vi "Initialise All Modbus Devices.vi"(8 "error in (no error)":errorcluster, 11 "Data Cluster in":T1 {"Flexi-Flow Devices"."Control State"."Control Mode" items=["Bus/RS232"=0, "FLOW-BUS slave"=2, "Valve close"=3, "Controller idle"=4, "Setpoint 100%"=7, "Valve fully open"=8, "Calibration mode"=9, "Setpoint 0%"=12, "RS232"=18, "Valve steering"=20, "Valve safe state"=22]}) -> (0 "error out":errorcluster, 3 "Data Cluster out":T1 {"Flexi-Flow Devices"."Control State"."Control Mode" items=["Bus/RS232"=0, "FLOW-BUS slave"=2, "Valve close"=3, "Controller idle"=4, "Setpoint 100%"=7, "Valve fully open"=8, "Calibration mode"=9, "Setpoint 0%"=12, "RS232"=18, "Valve steering"=20, "Valve safe state"=22]})   [LabVIEW 2025]
uses:
  phlair-shared-libraries/Modbus Flexi-Flow API/Bronkhorst Flexi-Flow ModbusTCP API.lvlib
  phlair-shared-libraries/Modbus Flexi-Flow API/Control Function Values--enum.ctl
  Modbus Flexi-Flow Controls--cluster.ctl
  FlexiFlowInterface.lvlib
  <vilib>/Plasmionique/MB Master/MB_Master_TCP/MB_Master_TCP.lvclass
  Modbus Flexi-Flow Measure State--cluster.ctl
  Modbus Flexi-Flow State--cluster.ctl
  Module Data--cluster.ctl
  phlair-shared-libraries/Modbus Flexi-Flow API/Control Mode--enum.ctl
  Device Type--enum.ctl
  Modbus TCP Connection Settings--cluster.ctl
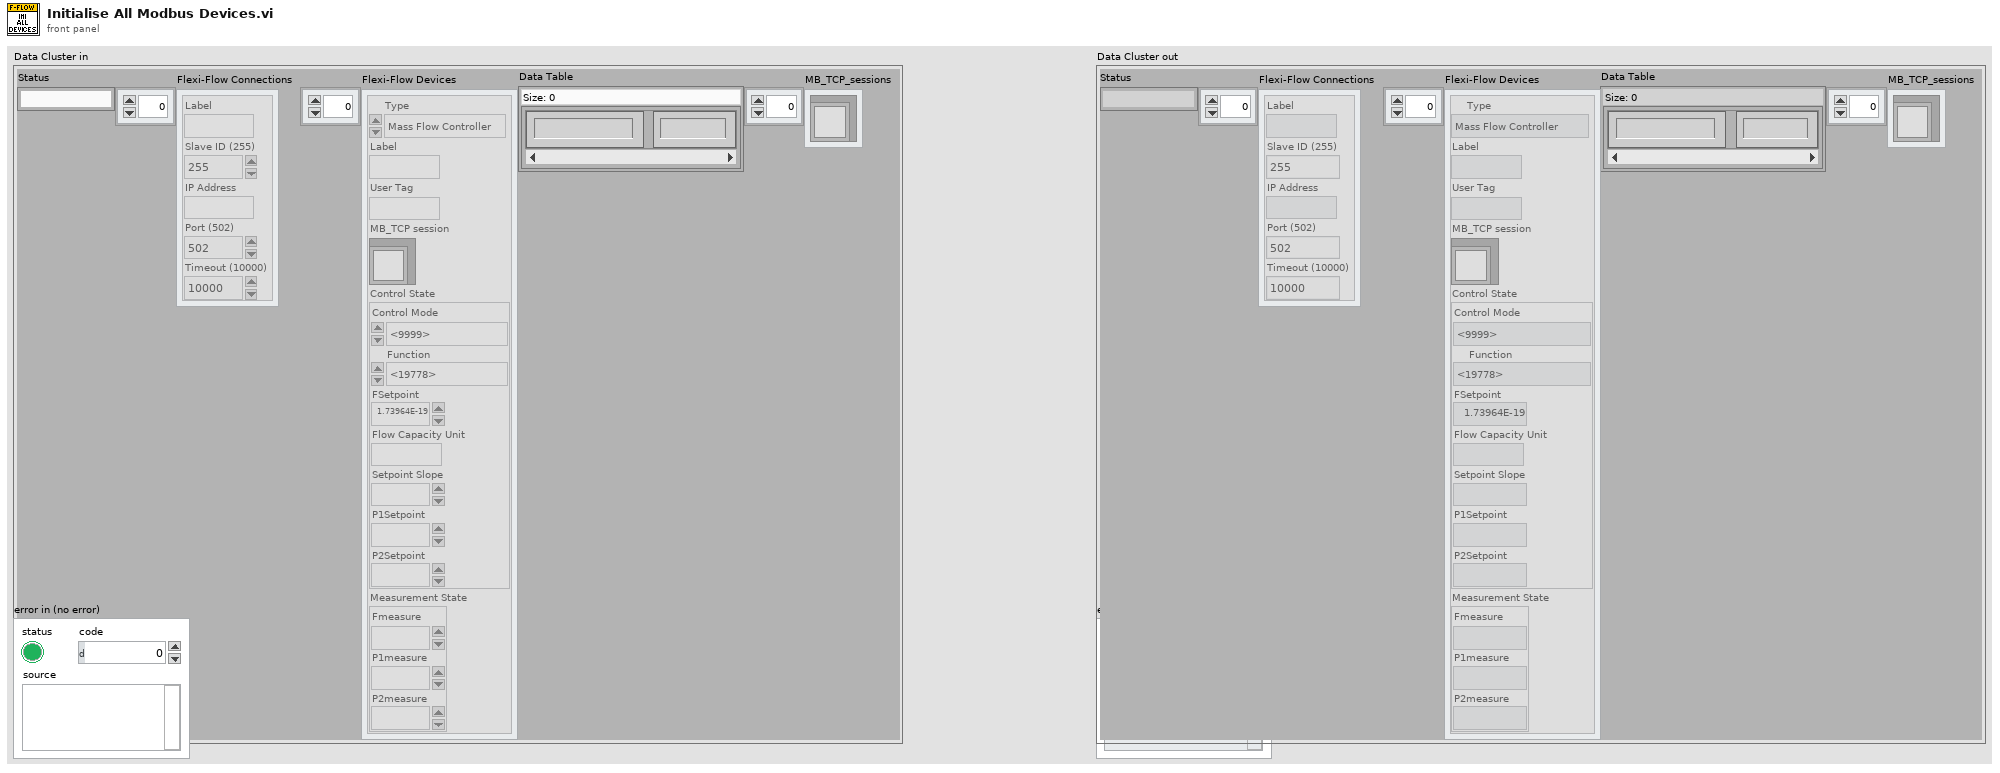
[diagram p1: front panel]
types:
  T1 = typedef "FlexiFlowInterface.lvlib/Module Data--cluster.ctl" = cluster{"Status":string, "Flexi-Flow Connections":T2[], "Flexi-Flow Devices":T3[], "Data Table":map{string, dbl}, "MB_TCP_sessions":refnum<class "MB_Master_TCP.lvclass">[]}
  T2 = typedef "FlexiFlowInterface.lvlib/Modbus TCP Connection Settings--cluster.ctl" = cluster{"Label":string, "Slave ID (255)":u8, "IP Address":string, "Port (502)":u16, "Timeout (10000)":i32}
  T3 = typedef "FlexiFlowInterface.lvlib/Modbus Flexi-Flow State--cluster.ctl" = cluster{"Type":T4, "Label":string, "User Tag":string, "MB_TCP session":refnum<class "MB_Master_TCP.lvclass">, "Control State":T5, "Measurement State":T8}
  T4 = typedef "FlexiFlowInterface.lvlib/Device Type--enum.ctl" = enum16{"Mass Flow Controller", "Mass Flow Meter"}
  T5 = typedef "FlexiFlowInterface.lvlib/Modbus Flexi-Flow Controls--cluster.ctl" = cluster{"Control Mode":T6, "Function":T7, "FSetpoint":sgl, "Flow Capacity Unit":string, "Setpoint Slope":u16, "P1Setpoint":sgl, "P2Setpoint":sgl}
  T6 = typedef "Bronkhorst Flexi-Flow ModbusTCP API.lvlib/Control Mode--enum.ctl" = u16
  T7 = typedef "Bronkhorst Flexi-Flow ModbusTCP API.lvlib/Control Function Values--enum.ctl" = enum16{"Flow", "Upstream pressure", "Downstream pressure", "Flow with upstream pressure limit", "Flow with downstream pressure limit", "Upstream pressure with flow limit", "Downstream pressure with flow limit"}
  T8 = typedef "FlexiFlowInterface.lvlib/Modbus Flexi-Flow Measure State--cluster.ctl" = cluster{"Fmeasure":dbl, "P1measure":sgl, "P2measure":sgl}
  T9 = typedef "FlexiFlowInterface.lvlib/Modbus Flexi-Flow State--cluster.ctl" = cluster{"MB_TCP session":refnum<class "MB_Master_TCP.lvclass">, "Control State":T10, "Measurement State":T8}
  T10 = typedef "FlexiFlowInterface.lvlib/Modbus Flexi-Flow Controls--cluster.ctl" = cluster{"Function":T7, "Control SP":sgl}
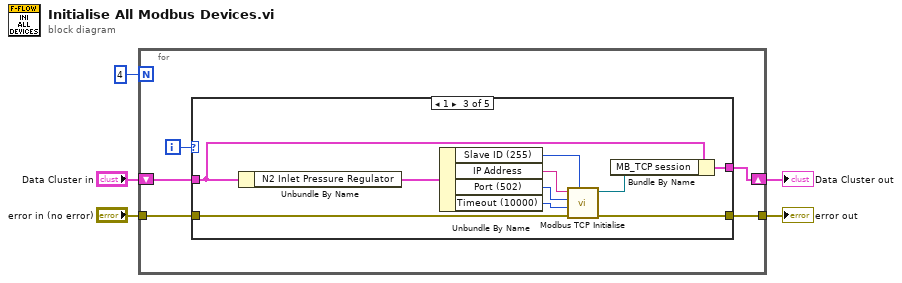
[diagram p0: block diagram]
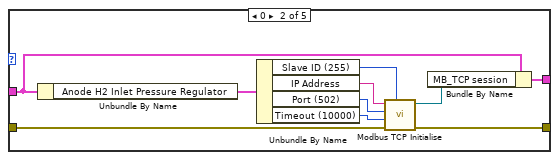
[diagram p3: hidden frame]
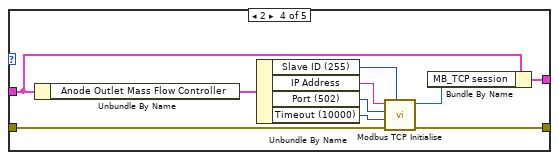
[diagram p4: hidden frame]
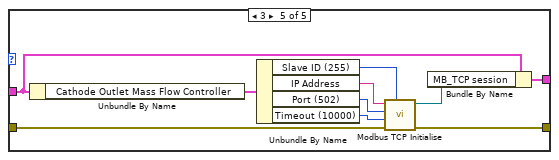
[diagram p5: hidden frame]
diagram:
  n1 = for {
    N: 4 -> [_]
    shift-right: [w9] -> w4
    shift-left: "Data Cluster in" -> [w8]
    tunnel: "error in (no error)" -> [w7]
    tunnel: [w10] -> w5
    i -> [w6]
    n2 = case shown="1" w6 {
      tunnel: [w12 w21 w31 w41 w51] -> w10
      tunnel: [w11 w20 w30 w40 w50] -> w9
      tunnel: w8 -> [w11 w17 w24 w34 w44]
      tunnel: w7 -> [w12 w19 w29 w39 w49]
      frame Default {
      }
      frame 0 {
        n3 = Unbundle By Name(w17) -> ("Anode H2 Inlet Pressure Regulator"=w18:T9)
        n4 = Unbundle By Name(w18) -> ("Slave ID (255)"=w13:u8, "IP Address"=w16:string, "Port (502)"=w15:u16, "Timeout (10000)"=w14:i32)
        n5 = call "Modbus TCP Initialise.vi"("Slave ID (255)"=w13, "error in (no error)"=w19, "Timeout (10000)"=w14, "Port (502)"=w15, "IP Address"=w16) -> ("error out"=w21:errorcluster, "MB_TCP session"=w22:refnum<class "MB_Master_TCP.lvclass">)  [unwired: 5 in]
        n6 = Bundle By Name(cluster=w17, "MB_TCP session"=w22) -> (w20:T1)
      }
      frame 1 {
        n7 = Unbundle By Name(w24) -> ("N2 Inlet Pressure Regulator"=w23:T9)
        n8 = Unbundle By Name(w23) -> ("Slave ID (255)"=w26:u8, "IP Address"=w25:string, "Port (502)"=w27:u16, "Timeout (10000)"=w28:i32)
        n9 = call "Modbus TCP Initialise.vi"("Slave ID (255)"=w26, "error in (no error)"=w29, "Timeout (10000)"=w28, "Port (502)"=w27, "IP Address"=w25) -> ("error out"=w31:errorcluster, "MB_TCP session"=w32:refnum<class "MB_Master_TCP.lvclass">)  [unwired: 5 in]
        n10 = Bundle By Name(cluster=w24, "MB_TCP session"=w32) -> (w30:T1)
      }
      frame 2 {
        n11 = Unbundle By Name(w34) -> ("Anode Outlet Mass Flow Controller"=w33:T9)
        n12 = Unbundle By Name(w33) -> ("Slave ID (255)"=w36:u8, "IP Address"=w35:string, "Port (502)"=w37:u16, "Timeout (10000)"=w38:i32)
        n13 = call "Modbus TCP Initialise.vi"("Slave ID (255)"=w36, "error in (no error)"=w39, "Timeout (10000)"=w38, "Port (502)"=w37, "IP Address"=w35) -> ("error out"=w41:errorcluster, "MB_TCP session"=w42:refnum<class "MB_Master_TCP.lvclass">)  [unwired: 5 in]
        n14 = Bundle By Name(cluster=w34, "MB_TCP session"=w42) -> (w40:T1)
      }
      frame 3 {
        n15 = Unbundle By Name(w44) -> ("Cathode Outlet Mass Flow Controller"=w43:T9)
        n16 = Unbundle By Name(w43) -> ("Slave ID (255)"=w46:u8, "IP Address"=w45:string, "Port (502)"=w47:u16, "Timeout (10000)"=w48:i32)
        n17 = call "Modbus TCP Initialise.vi"("Slave ID (255)"=w46, "error in (no error)"=w49, "Timeout (10000)"=w48, "Port (502)"=w47, "IP Address"=w45) -> ("error out"=w51:errorcluster, "MB_TCP session"=w52:refnum<class "MB_Master_TCP.lvclass">)  [unwired: 5 in]
        n18 = Bundle By Name(cluster=w44, "MB_TCP session"=w52) -> (w50:T1)
      }
    }
  }
  "error out" <- w5
  "Data Cluster out" <- w4
